vi "查询启动项.vi"(8 "error in (no error)":errorcluster caption="错误输入（无错误）") -> (0 "error out":errorcluster caption="错误输出", 3 "包含启动项":bool)   [LabVIEW 2016]
uses:
  <vilib>/registry/registry.llb/Registry RtKey.ctl
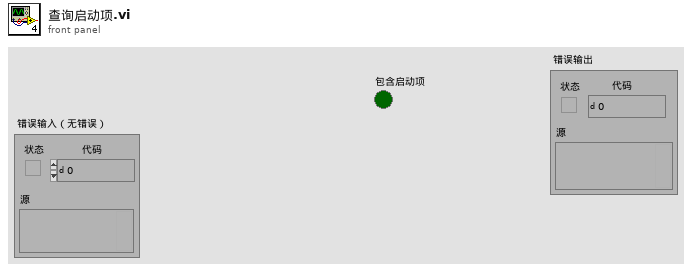
[diagram p1: front panel]
types:
  T1 = typedef "Registry RtKey.ctl" = enum32{"HKEY_CLASSES_ROOT", "HKEY_CURRENT_USER", "HKEY_LOCAL_MACHINE", "HKEY_USERS", "HKEY_PERFORMANCE_DATA", "HKEY_CURRENT_CONFIG", "HKEY_DYN_DATA"}
  T2 = typedef "Registry refnum.ctl" = refnum<k1>
  T3 = cluster{"numValues":i32, "maxValueNameLen":i32, "maxValueDataLen":i32}
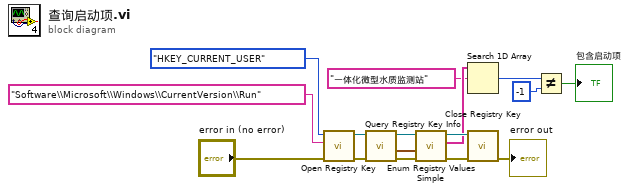
[diagram p0: block diagram]
diagram:
  n1 = call <vilib>:"Open Registry Key.vi"("error in (no error)"="error in (no error)", "subkey"="Software\\Microsoft\\Windows\\CurrentVersion\\Run", "root key (HKEY_LOCAL_MACHINE)"=Registry_RtKey."HKEY_CURRENT_USER") -> ("error out"=w12:errorcluster, "refnum out"=w13:T2)  [unwired: 7 in]
  n2 = call <vilib>:"Query Registry Key Info.vi"("error in (no error)"=w12, "refnum"=w13) -> ("error out"=w9:errorcluster, "value info"=w10:T3, "refnum out"=w11:T2)  [unwired: 5 in, 2 out]
  n3 = call <vilib>:"Enum Registry Values Simple.vi"("error in (no error)"=w9, "value info"=w10, "refnum"=w11) -> ("error out"=w7:errorcluster, "values"=w6:string[], "refnum out"=w8:T2)  [unwired: 3 in, 3 out]
  n4 = Search 1D Array(1D array=w6, element="一体化微型水质监测站" ("元素")) -> (index of element=w5:i32)  [unwired: 1 in]
  n5 = call <vilib>:"Close Registry Key.vi"("error in (no error)"=w7, "refnum"=w8) -> ("error out"=→"error out":errorcluster)  [unwired: 5 in]
  n6 = Not Equal?(x=w5, y=-1) -> (x != y?=→"包含启动项":bool)
